vi "FilePermisionEveryone.vi"(8 "error in (no error)":errorcluster, 11 "Path":path) -> (0 "error out":errorcluster, 1 "return code":i32, 2 "standard error":string, 3 "standard output":string)   [LabVIEW 2015]
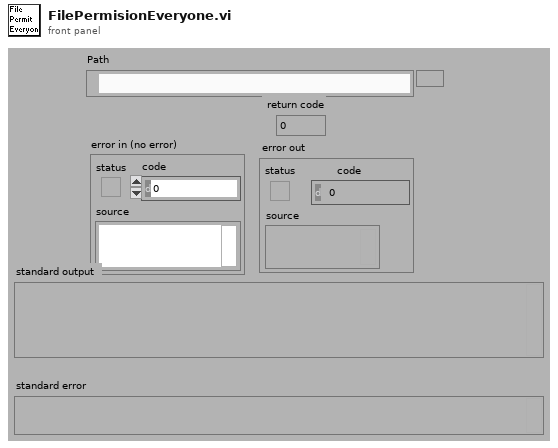
[diagram p1: front panel]
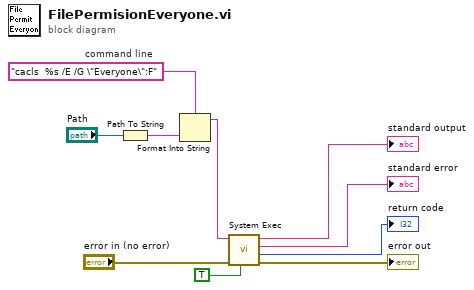
[diagram p0: block diagram]
diagram:
  w6 = "cacls  %s /E /G \"Everyone\":F"  # command line
  n1 = Path To String(path="Path") -> (string=w7:string)
  n2 = Format Into String(format string=w6, w7) -> (resulting string=w5:string)  [unwired: 2 in, 1 out]
  n3 = call <vilib>:"System Exec.vi"("run minimized? (F)"=TRUE, "error in (no error)"="error in (no error)", "command line"=w5) -> ("error out"=→"error out":errorcluster, "return code"=→"return code":i32, "standard error"=→"standard error":string, "standard output"=→"standard output":string)  [unwired: 3 in, 2 out]
